vi "OpenScan-20170126-Host.vi"() -> ()   [LabVIEW 2015]
uses:
  <vilib>/FPGAPlugInAG/PXIe-7972R/niLvFpga_Open_PXIe-7972R.vi
  <vilib>/rvi/interface/common/dynamic/niFpgaDynamicAddResources.vi
  <vilib>/FPGAPlugInAG/Dynamic/niLvFpga_Reset_Dynamic.vi
  <vilib>/FPGAPlugInAG/Dynamic/niLvFpga_Run_Dynamic.vi
  <vilib>/Utility/error.llb/Error Cluster From Error Code.vi
  <vilib>/rvi/errors/niLvFpgaAdjustHostInterfaceError.vi
  <vilib>/FPGAPlugInAG/Dynamic/niLvFpga_Close_Dynamic.vi
  <vilib>/rvi/interface/nirviOpenFPGA/nirviOpenFPGA.xnode
  FPGA Bitfiles/OpenScan-2017030_FPGATarget_OpenScan-packedD_9efvn6-7f3g.lvbitx
  OpenScan-packed DRAM-FPGA.vi
  <vilib>/rvi/interface/nirviMethod/nirviMethod.xnode
  <vilib>/rvi/interface/nirviReadWriteControl/nirviReadWriteControl.xnode
  <vilib>/rvi/interface/nirviCloseFPGA/nirviCloseFPGA.xnode
  <vilib>/rvi/errors/niLvFpgaMergeErrorWithErrorCode.vi
  <vilib>/FPGAPlugInAG/Dynamic/niLvFpga_ReadFifo_Dynamic.vi
  <vilib>/FPGAPlugInAG/Dynamic/niLvFpga_StopFifo_Dynamic.vi
  NiFpgaLv.dll
  <vilib>/rvi/interface/Simulation/niFpgaSimulationCallBeginRW.vi
  <vilib>/FPGAPlugInAG/Dynamic/niLvFpga_WriteFifo_Dynamic.vi
panel:
  out "Kalman done?":bool
  in  "Save Kalman result?":bool
  out "Scanning?":bool
  out "FPGA VI Reference Out":refnum<k20>
  out "Total frames":u32
  out "Kalman done":u32
  in  "Kalman averaging factor":u32=1
  out "Frame address_indicator":u32
  out "Frame Galvo signal write done?":bool
  in  "?":bool
  out "Resolution":i32
  out "Kalman averaged image":T1(plugin-control)
  out "Kalman gain":fxp<+,32,0>=0.3333333332557231 format="%.32g"
  out "Frame averaged?":bool
  in  "Filter gain":fxp<+,16,0>=0.9999847412109375 format="%.16g"
  in  "File name base":string="Imaing data1112-"
  in  "Save image?":bool
  out "error out 3":errorcluster
  out "Original Image":T1(plugin-control)
  out "Elements Remaining":u32
  out "Frames done":u32=2
  out "data size":i32
  in  "Frame retrace time(ms)":u32=1000
  in  "Imaging data base path":path=path "C:/Users/LOCI/Documents/openscan/openscan/Imaging data"
  in  "Imaging mode":i16(ring)=2 items=["Grab, single frame", "Loop, finite frames", "Focus, infinite frames"]
  in  "Num of frames":i32=214758367
  in  "ZoomY":dbl=0.8 step=0.1
  in  "Zoom X":sgl=0.8 step=0.1
  out "Total data size":i32
  out "min index(es)":i32=-1
  out "min value":u16
  out "max index(es)":i32=-1
  out "max value":u16
  out "error out 2":errorcluster
  out "Samples acquired":u32=262144
  out "Acquisition finish?":bool
  out "Frame imaging data averaged?":bool=TRUE
  in  "Pixel pulse_initial delay(ticks)":i32=1
  out "Waveform info out":T2={"Frame address"=512000, "Write DRAM done?"=TRUE, "Waveform output finish?"=FALSE, "Request address"=512000}
  in  "Galvo signal data file path":T3={"file path_Y Galvo (use dialog)"=path "", "file path_X Galvo (use dialog)"=path "C:/Users/LOCI/Documents/MATLAB/ScanImage/scanner signal/xx.txt"}
  in  "Waveform info in":T2
  in  "Trigger controls":T4={"Pixel clock_pulse width ratio"=0.7, "Resolution"=512, "Num of undershoot"=50} {"Pixel clock_pulse width ratio" step=0.1}
  in  "Waveform controls":T5={"Scan rate(MHz)"=0.5, "Elements per line"=1000} {"Scan rate(MHz)" step=0.1}
  out "Numeric Control":i32=40162
  out "Galvo Y":u16[](graph)
  out "Frame time":dbl=9.152740529214498
  out "error out":errorcluster
  out "Galvo X":u16[](graph)
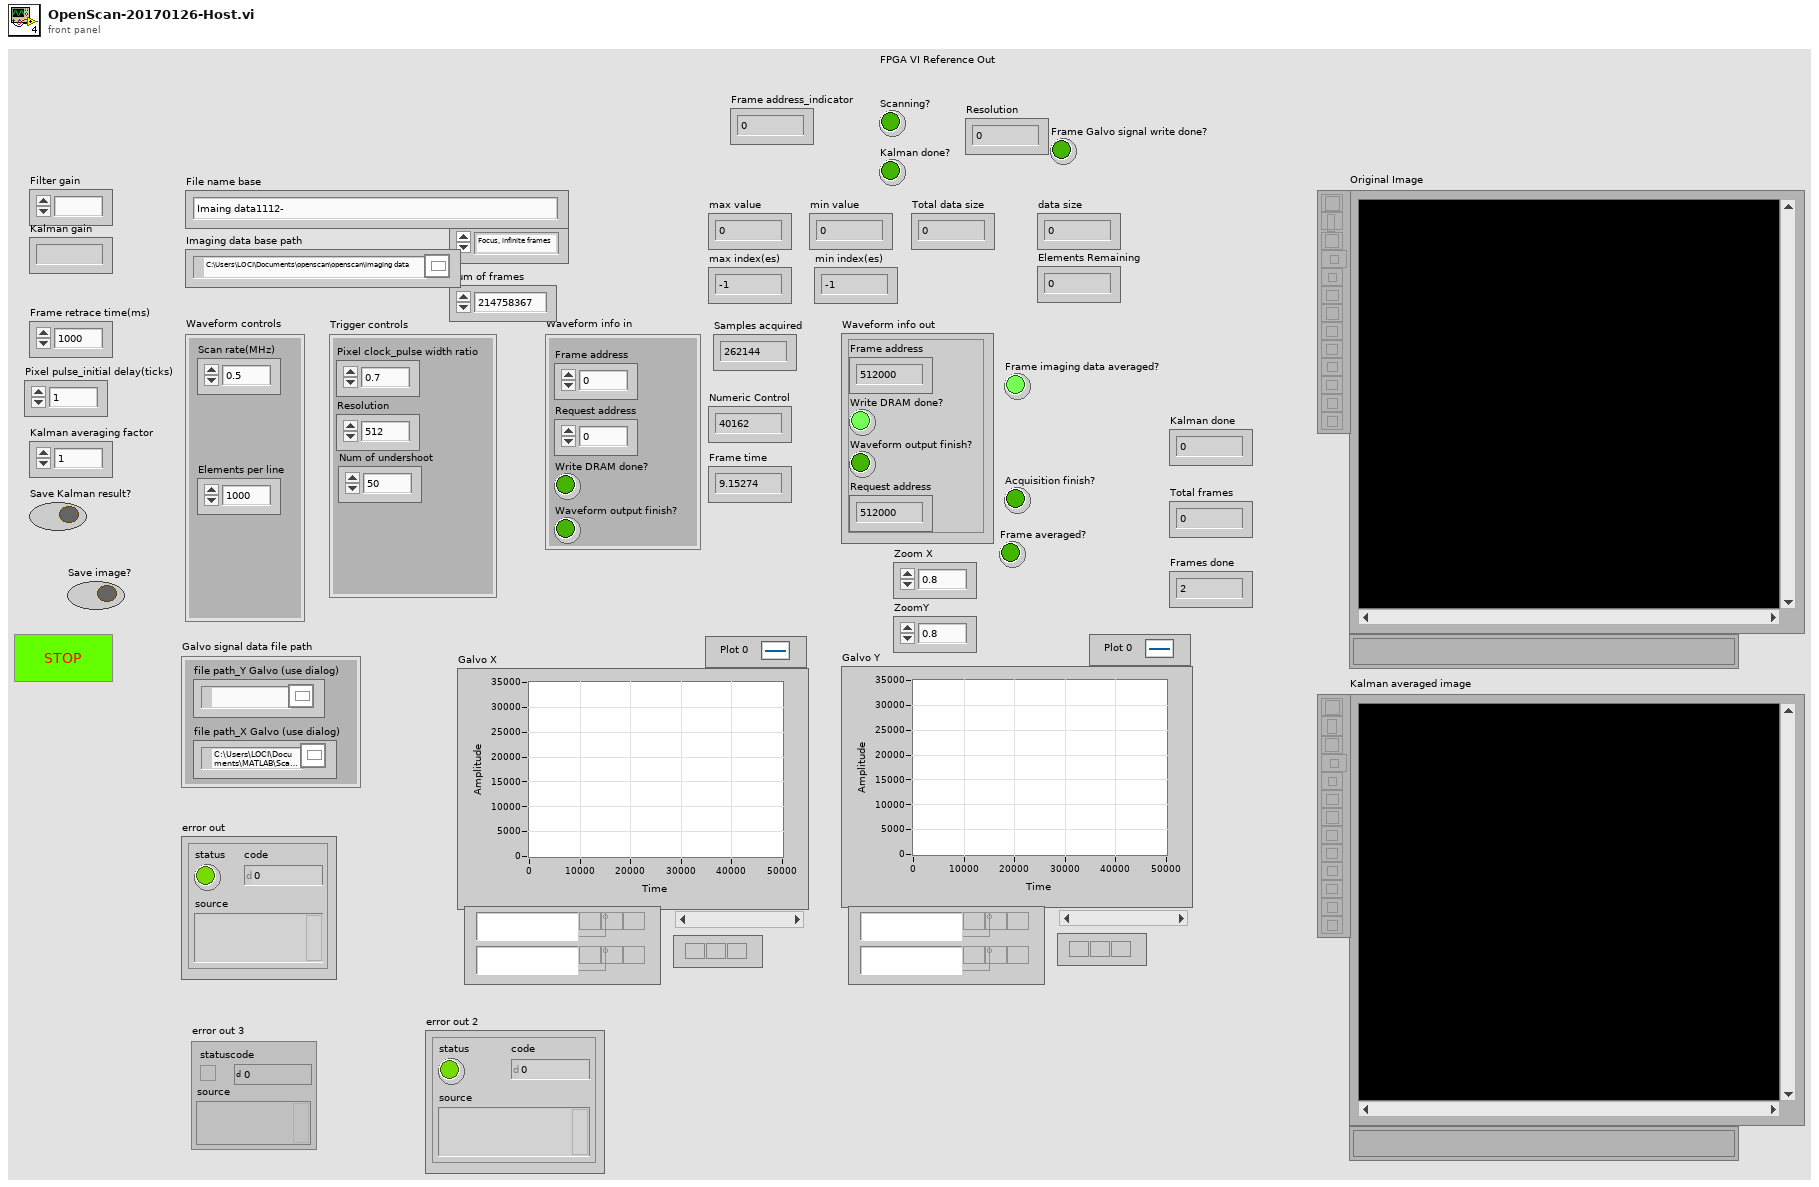
[diagram p1: front panel]
types:
  T1 = typedef "IMAQ Image.ctl" = refnum<image>
  T2 = cluster{"Frame address":u32, "Write DRAM done?":bool, "Waveform output finish?":bool, "Request address":u32}
  T3 = cluster{"file path_Y Galvo (use dialog)":path, "file path_X Galvo (use dialog)":path}
  T4 = cluster{"Pixel clock_pulse width ratio":dbl, "Resolution":i32, "Num of undershoot":i32}
  T5 = cluster{"Scan rate(MHz)":dbl, "Elements per line":u32}
  T6 = enum16{"open", "replace", "create", "open or create", "replace or create", "replace or create with confirmation"}
  T7 = typedef "Image Type" = u32
  T8 = typedef "LVDateTimeRec.ctl" = cluster{"fractional second":dbl, "second":i32, "minute":i32, "hour":i32, "day of month":i32, "month":i32, "year":i32, "day of week":i32, "day of year":i32, "DST":i32}
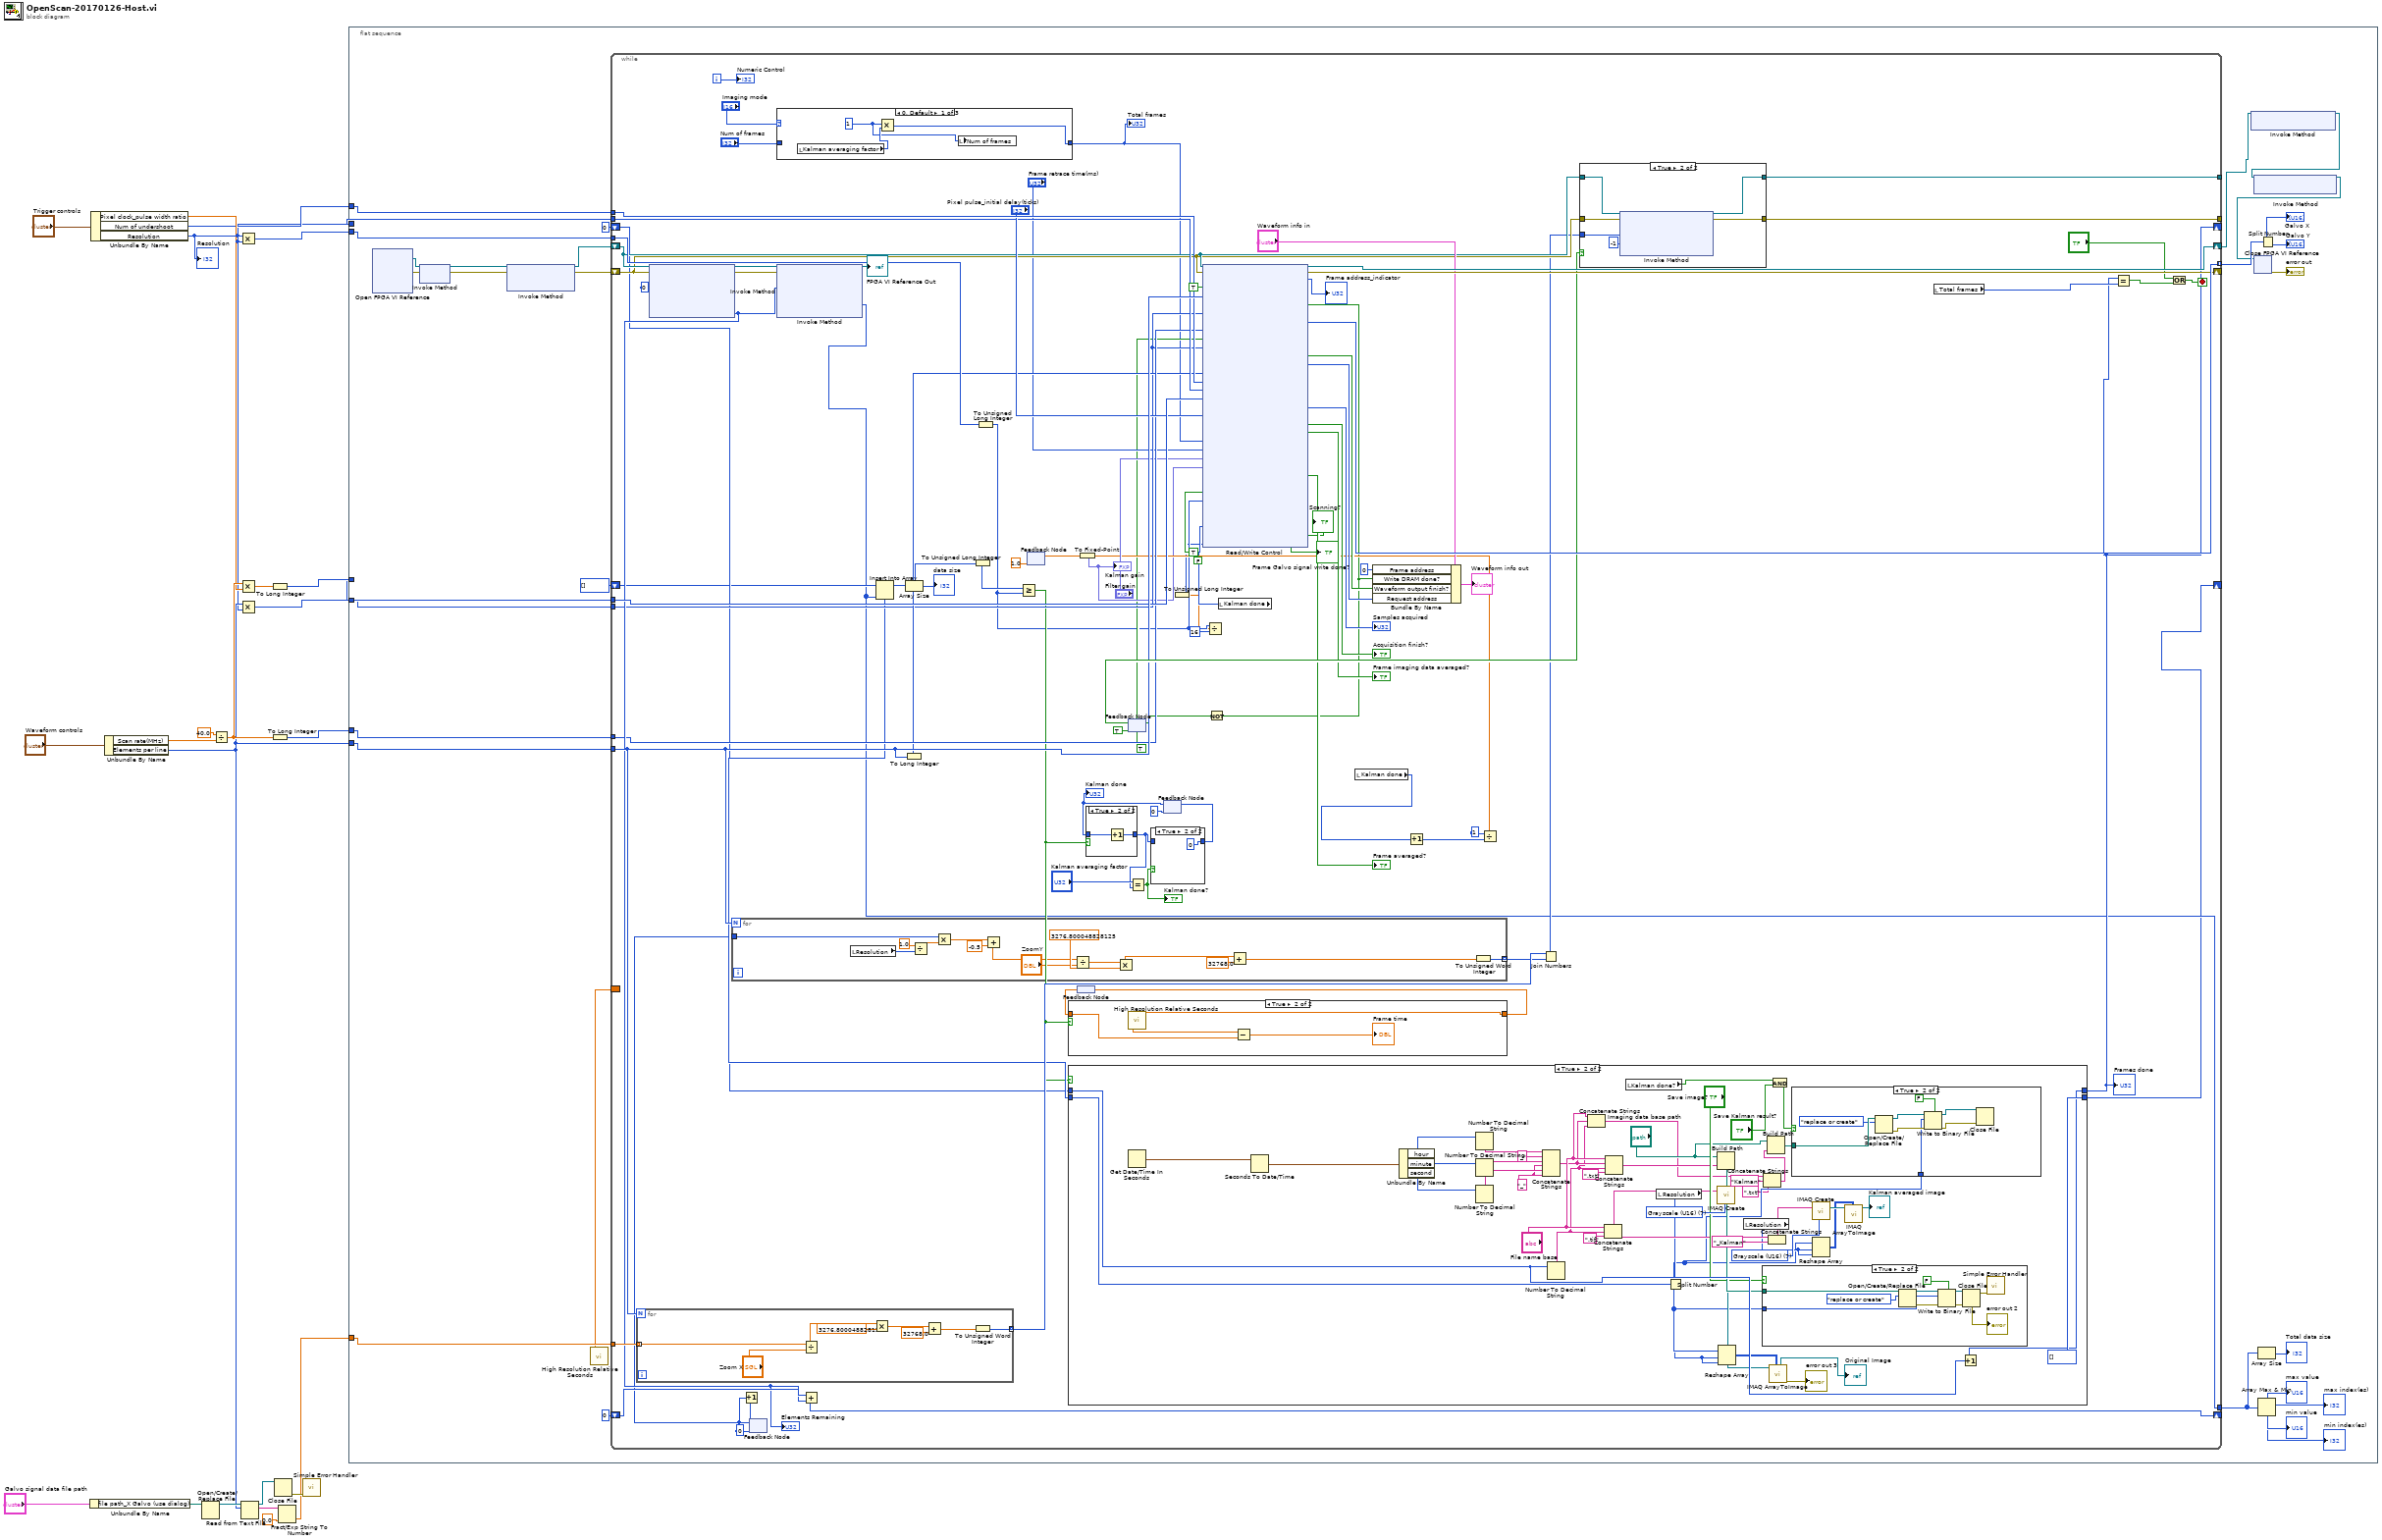
[diagram p0: block diagram]
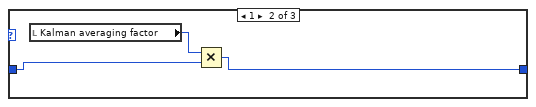
[diagram p5: hidden frame]
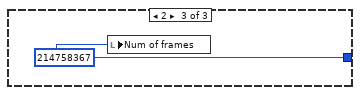
[diagram p6: hidden frame]
diagram:
  n1 = Unbundle By Name("Galvo signal data file path") -> ("file path_X Galvo (use dialog)"=w8:path)
  n2 = Unbundle By Name("Trigger controls") -> ("Pixel clock_pulse width ratio"=w6:dbl, "Num of undershoot"=w5:i32, "Resolution"=w2:i32)
  "Resolution" <- w2
  n3 = Unbundle By Name("Waveform controls") -> ("Scan rate(MHz)"=w10:dbl, "Elements per line"=w3:u32)
  n4 = Open/Create/Replace File(file path (use dialog)=w8) -> (refnum out=w19:refnum<file>)  [unwired: 5 in, 2 out]
  n5 = Divide(x=40.0 ("y"), y=w10) -> (x/y=w14:dbl)
  n6 = Multiply(x=w2, y=w2) -> (x*y=w4:i32)
  n7 = Multiply(x=w14, y=w6) -> (x*y=w13:dbl)
  n8 = Multiply(x=w3, y=w2) -> (x*y=w1:u32)
  n9 = Read from Text File(file (use dialog)=w19, count=w3) -> (refnum out=w20:refnum<file>, text=w21:string[])  [unwired: 2 in, 2 out]
  n10 = To Long Integer(number=w13) -> (32bit integer=w12:i32)
  n11 = To Long Integer(number=w14) -> (32bit integer=w16:i32)
  n12 = Close File(refnum=w20) -> (error out=w18:errorcluster)  [unwired: 1 in, 1 out]
  n13 = Fract/Exp String To Number(string=w21, default (0 dbl)=sgl 0.0 ("default (0 DBL)")) -> (number=w17:sgl[])  [unwired: 2 in, 1 out]
  n14 = call <vilib>:"Simple Error Handler.vi"("error in (no error)"=w18) -> ()  [unwired: 4 in, 5 out]
  n15 = flat-sequence {
    tunnel: w3 -> [w53]
    tunnel: w17 -> [w52]
    tunnel: w16 -> [w51]
    tunnel: w12 -> [w50]
    tunnel: w1 -> [w49]
    tunnel: w2 -> [w46]
    tunnel: w5 -> [w48]
    tunnel: w4 -> [w47]
    frame #0 {
      n16 = xnode "Open FPGA VI Reference"() -> ("FPGA VI Reference Out"=w40:refnum<k20>, "error out"=w39:errorcluster)  [unwired: 2 in]
      n17 = xnode "Invoke Method"("FPGA VI Reference In"=w40, "error in"=w39) -> ("FPGA VI Reference Out"=w27:refnum<k20>, "error out"=w26:errorcluster)
      n18 = xnode "Invoke Method"("FPGA VI Reference In"=w27, "error in"=w26) -> ("FPGA VI Reference Out"=w38:refnum<k20>, "error out"=w37:errorcluster)  [unwired: 1 in]
      n19 = call <vilib>:"High Resolution Relative Seconds.vi"() -> ("relative seconds"=w28:dbl)
      n20 = while {
        tunnel: w53 -> [w133]
        shift-right: [w136] -> w25
        shift-left: w38 -> [w122]
        shift-right: [w135] -> _
        shift-left: w37 -> [w121]
        tunnel: w52 -> [w141]
        tunnel: [w138] -> w44 mode=indexing
        tunnel: w51 -> [w114]
        tunnel: w50 -> [w132]
        tunnel: w49 -> [w109]
        tunnel: w48 -> [w131]
        tunnel: w47 -> [w126]
        tunnel: w46 -> [w125]
        tunnel: [w60] -> w32
        shift-right: [w115] -> _
        shift-left: u32 0 ("Number of Elements") -> [w117]
        shift-right: [w58] -> _
        shift-left: u32[] [] ("array") -> [w97]
        shift-right: [w74] -> _
        shift-left: u32 0 ("Number of Elements") -> [w107]
        tunnel: [w101] -> _
        border: w28 -> [_]
        tunnel: [w75] -> _
        i -> [w111]
        stop <- w77 stop-if-true
        (unwired) FALSE ("Ready to Scan")
        n21 = for {
          N: w133 -> [_]
          tunnel: [w239] -> w140 mode=indexing
          tunnel: w141 -> [w233] mode=indexing
          n22 = Divide(x=w233, y="Zoom X") -> (x/y=w234:sgl)
          n23 = Multiply(x=w234, y=sgl 3276.8) -> (x*y=w237:sgl)
          n24 = Add(x=w237, y=sgl 32768.0) -> (x+y=w235:sgl)
          n25 = To Unsigned Word Integer(number=w235) -> (unsigned 16bit integer=w239:u16)
        }
        n26 = xnode "Invoke Method"("FPGA VI Reference In"=w122, "error in"=w121, "Number of Elements"=u32 0) -> ("FPGA VI Reference Out"=w119:refnum<k20>, "error out"=w118:errorcluster, "Elements Remaining"=w116:u32)  [unwired: 1 in, 1 out]
        "Elements Remaining" <- w116
        n27 = feedback #1(0 ("dimension size")) -> (w86:i32)
        n28 = for {
          N: w133 -> [_]
          tunnel: [w253] -> w139 mode=indexing
          tunnel: w86 -> [w241]
          n29 = local read "Resolution"() -> (w240:i32)
          n30 = Divide(x=1.0, y=w240) -> (x/y=w248:dbl)
          n31 = Multiply(x=w241, y=w248) -> (x*y=w247:dbl)
          n32 = Add(x=w247, y=-0.5) -> (x+y=w244:dbl)
          n33 = Divide(x=w244, y="ZoomY") -> (x/y=w245:dbl)
          n34 = Multiply(x=w245, y=sgl 3276.8) -> (x*y=w251:dbl)
          n35 = Add(x=w251, y=sgl 32768.0) -> (x+y=w242:dbl)
          n36 = To Unsigned Word Integer(number=w242) -> (unsigned 16bit integer=w253:u16)
        }
        n37 = Increment(x=w86) -> (x+1=w88:i32)
        n38 = feedback-in #1(w88) -> ()
        n39 = case shown="0, Default" "Imaging mode" {
          tunnel: "Num of frames" -> [_ w156 _]
          tunnel: [w152 w154 w157] -> w65
          frame 0, Default {
            w151 = 1 ("Num of frames")
            n40 = local read "Kalman averaging factor"() -> (w153:u32)
            n41 = Multiply(x=w151, y=w153) -> (x*y=w152:u32)
            n42 = local write "Num of frames"(w151) -> ()
          }
          frame 1 {
            n43 = local read "Kalman averaging factor"() -> (w155:u32)
            n44 = Multiply(x=w155, y=w156) -> (x*y=w154:u32)
          }
          frame 2 {
            w157 = 214758367 ("Num of frames")
            n45 = local write "Num of frames"(w157) -> ()
          }
        }
        "Total frames" <- w65
        n46 = xnode "Invoke Method"("FPGA VI Reference In"=w119, "error in"=w118, "Number of Elements"=w116) -> ("FPGA VI Reference Out"=→"FPGA VI Reference Out":refnum<k20>, "Data"=w60:u32[])  [unwired: 1 in, 2 out]
        n47 = Add(x=w117, y=w116) -> (x+y=w115:u32)
        n48 = Insert Into Array(array=w97, new element=w60) -> (w108:u32[])  [unwired: 1 in]
        n49 = To Long Integer(number=w133) -> (32bit integer=w113:i32)
        n50 = Array Size(array=w108) -> (size(s)=w110:i32)
        "data size" <- w110
        n51 = To Unsigned Long Integer(number=w110) -> (unsigned 32bit integer=w98:u32)
        n52 = To Unsigned Long Integer(number=w126) -> (unsigned 32bit integer=w57:u32)
        n53 = Greater Or Equal?(x=w98, y=w57) -> (x >= y?=w67:bool)
        n54 = feedback #2(1.0) -> (w92:dbl)
        n55 = case shown="True" w67 {
          tunnel: w108 -> [w159 w201]
          tunnel: [w159 u32[] [] ("array")] -> w58
          tunnel: w107 -> [w158 w205]
          tunnel: [w158 w204] -> w74
          frame False {
          }
          frame True {
            w181 = T7 7 items=["Grayscale (U8)", "Grayscale (I16)", "Grayscale (SGL)", "Complex (CSG)", "RGB (U32)", "HSL (U32)", "RGB (U64)", "Grayscale (U16)"] ("Image Type")
            w184 = "_" ("string")
            w202 = T7 7 items=["Grayscale (U8)", "Grayscale (I16)", "Grayscale (SGL)", "Complex (CSG)", "RGB (U32)", "HSL (U32)", "RGB (U64)", "Grayscale (U16)"] ("Image Type")
            n56 = Get Date/Time In Seconds() -> (seconds since 1Jan1904=w194:timestamp)
            n57 = Seconds To Date/Time(time stamp (now)=w194) -> (date time rec=w193:T8)  [unwired: 1 in]
            n58 = Unbundle By Name(w193) -> ("hour"=w191:i32, "minute"=w192:i32, "second"=w186:i32)
            n59 = Number To Decimal String(number=w191) -> (decimal integer string=w190:string)  [unwired: 1 in]
            n60 = Number To Decimal String(number=w192) -> (decimal integer string=w188:string)  [unwired: 1 in]
            n61 = Number To Decimal String(number=w186) -> (decimal integer string=w185:string)  [unwired: 1 in]
            n62 = Concatenate Strings(w190, "_" ("string"), w188, w184, w185, w184) -> (w163:string)
            n63 = Number To Decimal String(number=w205) -> (decimal integer string=w162:string)  [unwired: 1 in]
            n64 = Concatenate Strings("File name base", w163, w162) -> (w161:string)
            n65 = Concatenate Strings("File name base", w162, ".tif" ("string")) -> (w180:string)
            n66 = Concatenate Strings("File name base", w163, w162, ".txt" ("string")) -> (w173:string)
            n67 = local read "Kalman done?"() -> (w166:bool)
            n68 = local read "Resolution"() -> (w174:i32)
            n69 = Split Number(x=w201) -> (hi(x)=w168:u16[], lo(x)=w183:u16[])
            n70 = Build Path(base path="Imaging data base path", name or relative path=w173) -> (appended path=w203:path)
            n71 = call "IMAQ Create"("Image Name"=w180, "Image Type"=w202) -> ("New Image"=w197:T1)  [unwired: 3 in, 1 out]
            n72 = Reshape Array(w183, w174, w174) -> (w196:u16[][])
            n73 = local read "Resolution"() -> (w175:i32)
            n74 = case shown="True" "Save image?" {
              tunnel: w203 -> [_ w219]
              tunnel: w183 -> [_ w217]
              frame False {
              }
              frame True {
                n75 = Open/Create/Replace File(file path (use dialog)=w219, operation (0:open)=T6."replace or create") -> (refnum out=w220:refnum<file>, error out=w222:errorcluster)  [unwired: 4 in, 1 out]
                n76 = Write to Binary File(file (use dialog)=w220, data=w217, error in=w222, 5:FALSE ("prepend array or string size? (T)")) -> (refnum out=w221:refnum<file>, error out=w223:errorcluster)  [unwired: 2 in, 1 out]
                n77 = Close File(refnum=w221, error in=w223) -> (error out=w218:errorcluster)  [unwired: 1 out]
                "error out 2" <- w218
                n78 = call <vilib>:"Simple Error Handler.vi"("error in (no error)"=w218) -> ()  [unwired: 4 in, 5 out]
              }
            }
            n79 = Concatenate Strings(w161, "Kalman" ("string"), ".txt" ("string")) -> (w170:string)
            n80 = Build Path(base path="Imaging data base path", name or relative path=w170) -> (appended path=w169:path)
            n81 = Concatenate Strings(w180, "_Kalman" ("string")) -> (w178:string)
            n82 = call "IMAQ ArrayToImage"("Image Pixels (U16)"=w196, "Image"=w197) -> ("error out"=→"error out 3":errorcluster, "Image Out"=→"Original Image":T1)  [unwired: 8 in]
            n83 = And(x=w166, y="Save Kalman result?") -> (x .and. y?=w165:bool)
            n84 = case shown="True" w165 {
              tunnel: w169 -> [_ w214]
              tunnel: w168 -> [_ w208]
              frame False {
              }
              frame True {
                n85 = Open/Create/Replace File(file path (use dialog)=w214, operation (0:open)=T6."replace or create") -> (refnum out=w211:refnum<file>, error out=w212:errorcluster)  [unwired: 4 in, 1 out]
                n86 = Write to Binary File(file (use dialog)=w211, data=w208, error in=w212, 5:FALSE ("prepend array or string size? (T)")) -> (refnum out=w210:refnum<file>, error out=w209:errorcluster)  [unwired: 2 in, 1 out]
                n87 = Close File(refnum=w210, error in=w209) -> ()  [unwired: 2 out]
              }
            }
            n88 = call "IMAQ Create"("Image Name"=w178, "Image Type"=w181) -> ("New Image"=w182:T1)  [unwired: 3 in, 1 out]
            n89 = Reshape Array(w168, w175, w175) -> (w176:u16[][])
            n90 = call "IMAQ ArrayToImage"("Image Pixels (U16)"=w176, "Image"=w182) -> ("Image Out"=→"Kalman averaged image":T1)  [unwired: 8 in, 1 out]
            n91 = Increment(x=w205) -> (x+1=w204:u32)
          }
        }
        "Frames done" <- w74
        n92 = feedback #3() -> (w90:dbl)
        n93 = case shown="True" w67 {
          tunnel: w90 -> [w147 w149]
          tunnel: [w147 w148] -> w89
          frame False {
          }
          frame True {
            n94 = call <vilib>:"High Resolution Relative Seconds.vi"() -> ("relative seconds"=w148:dbl)
            n95 = Subtract(x=w148, y=w149) -> (x-y=→"Frame time":dbl)
          }
        }
        n96 = feedback-in #3(w89) -> ()
        n97 = To Fixed-Point(number=w92) -> (fixed-point=w91:fxp<+,32,0>)  [unwired: 1 in]
        "Kalman gain" <- w91
        n98 = feedback #4(TRUE) -> (w134:bool)
        n99 = feedback #5(u32 0) -> (w66:u32)
        "Kalman done" <- w66
        n100 = case shown="True" w67 {
          tunnel: [w142 w144] -> w63
          tunnel: w66 -> [w142 w143]
          frame False {
          }
          frame True {
            n101 = Increment(x=w143) -> (x+1=w144:u32)
          }
        }
        n102 = Equal?(x="Kalman averaging factor", y=w63) -> (x = y?=w71:bool)
        "Kalman done?" <- w71
        n103 = case shown="True" w71 {
          tunnel: w63 -> [w145 _]
          tunnel: [w145 u32 0] -> w70
          frame False {
          }
          frame True {
          }
        }
        n104 = feedback-in #5(w70) -> ()
        n105 = Divide(x=w57, y=u32 16) -> (x/y=w55:dbl)
        n106 = To Unsigned Long Integer(number=w55) -> (unsigned 32bit integer=w54:u32)
        n107 = local read "Kalman done"() -> (w68:u32)
        n108 = xnode "Read/Write Control"("FPGA VI Reference In"=w122, "error in"=w121, "Write DRAM enable?"=TRUE, "max addr"=w133, "Num of elements"=w109, "Pixel time (tick)"=w114, "Write Frame Galvo signal?"=TRUE, "Total elements"=w109, "Elements per line"=w113, "Num of undershoot"=w131, "Resolution"=w125, "Pixel clock_pulse width(tick)"=w132, "Pixel pulse_initial delay"="Pixel pulse_initial delay(ticks)", "Number of frames"=w65, "Frame retrace time"="Frame retrace time(ms)", "Filter gain"="Filter gain", "Kalman gain"=w91, "Ready to Scan"=TRUE, "Samples per frame control"=w57, "Frame number"=w68, "Max DRAM address"=w54) -> ("FPGA VI Reference Out"=w136:refnum<k20>, "error out"=w135:errorcluster, "Frame address_indicator"=→"Frame address_indicator":u32, "Write DRAM done?"=w73:bool, "Data"=w138:u32, "Frame waveform output finish?"=w112:bool, "Request address"=w130:u32, "Samples acquired"=→"Samples acquired":u32, "Frame acquisition finish?"=→"Acquisition finish?":bool, "Frame imaging data averaged?"=→"Frame imaging data averaged?":bool, "Averaged image displayed?"=→"Frame averaged?":bool, "Frame Galvo signal write done?"=→"Frame Galvo signal write done?":bool, "Scanning?"=→"Scanning?":bool)  [unwired: 2 out]
        n109 = Not(x=w73) -> (.not. x?=w72:bool)
        n110 = feedback-in #4(w72) -> ()
        n111 = local read "Kalman done"() -> (w78:u32)
        n112 = Bundle By Name(cluster="Waveform info in", "Frame address"=u32 0, "Write DRAM done?"=w73, "Waveform output finish?"=w112, "Request address"=w130) -> (→"Waveform info out":T2)
        n113 = Increment(x=w78) -> (x+1=w96:u32)
        n114 = Divide(x=1, y=w96) -> (x/y=w94:dbl)
        n115 = feedback-in #2(w94) -> ()
        n116 = Join Numbers(hi=w140, lo=w139) -> ((hi.lo)=w80:u32[])
        n117 = case shown="True" w134 {
          tunnel: [w225 w231] -> w101
          tunnel: [w224 w230] -> w75
          tunnel: w80 -> [_ w228]
          tunnel: w122 -> [w225 w227]
          tunnel: w121 -> [w224 w226]
          frame False {
          }
          frame True {
            n118 = xnode "Invoke Method"("FPGA VI Reference In"=w227, "error in"=w226, "Data"=w228, "Timeout (ms)"=-1) -> ("FPGA VI Reference Out"=w231:refnum<k20>, "error out"=w230:errorcluster)  [unwired: 1 out]
          }
        }
        n119 = local read "Total frames"() -> (w104:u32)
        n120 = Equal?(x=w74, y=w104) -> (x = y?=w59:bool)
        n121 = Or(x="?", y=w59) -> (x .or. y?=w77:bool)
        "Numeric Control" <- w111
      }
      n122 = xnode "Invoke Method"("FPGA VI Reference In"=w25) -> ("FPGA VI Reference Out"=w24:refnum<k20>)  [unwired: 1 in, 1 out]
      n123 = xnode "Invoke Method"("FPGA VI Reference In"=w24) -> ("FPGA VI Reference Out"=w23:refnum<k20>)  [unwired: 1 in, 1 out]
      n124 = xnode "Close FPGA VI Reference"("FPGA VI Reference In"=w23) -> ("error out"=→"error out":errorcluster)  [unwired: 1 in]
      n125 = Array Size(array=w32) -> (size(s)=→"Total data size":i32)
      n126 = Array Max & Min(array=w32) -> (max value=→"max value":u32, max index (indices)=→"max index(es)":i32, min value=→"min value":u32, min index (indices)=→"min index(es)":i32)
      n127 = Split Number(x=w44) -> (hi(x)=→"Galvo X":u16[], lo(x)=→"Galvo Y":u16[])
    }
  }
